vi "IPC-Core-UDPModule.vi"(8 "error in":errorcluster, 9 "ErrorQRef":refnum<queue>, 10 "DataQRef":refnum<queue>, 11 "UdpQRef":refnum<queue>) -> (0 "错误输出":errorcluster)   [LabVIEW 2014]
uses:
  Configuration-Global.vi
panel:
  out "数值 2":i32
  out "数值":i32
  in  "开关":bool=TRUE
  out "Udp::Initialize":string
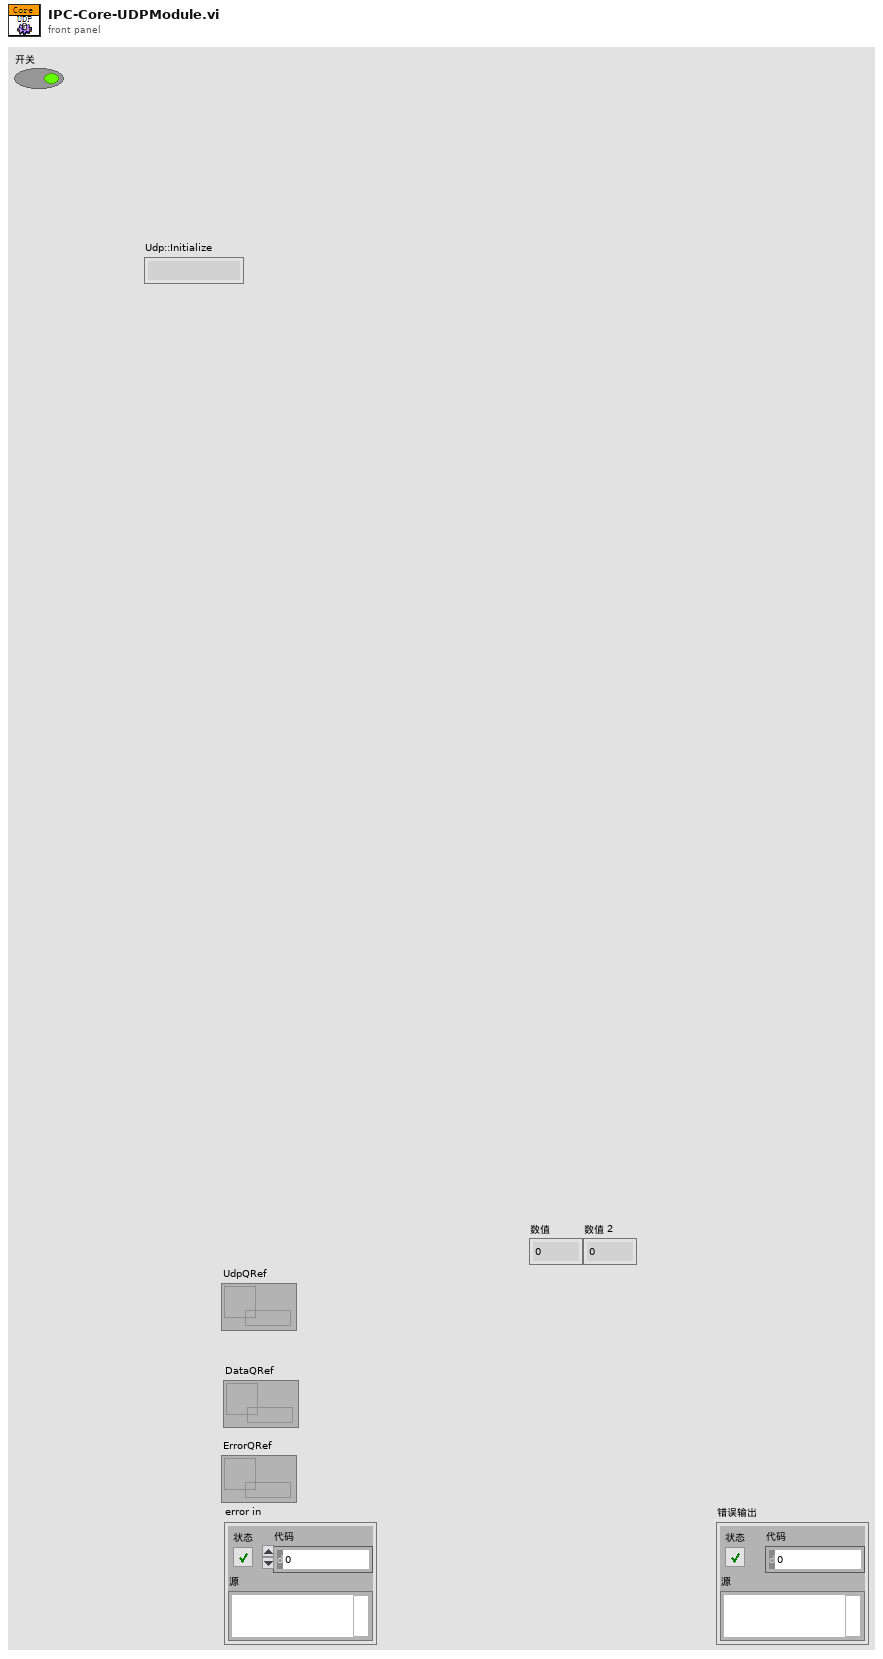
[diagram p1: front panel]
types:
  T1 = cluster{"时间":timestamp, "声发射":sgl[], "电涡流1":sgl[], "电涡流2":sgl[], "电涡流3":sgl[], "电涡流4":sgl[], "电涡流5":sgl[], "加速度1":sgl[], "加速度2":sgl[]}
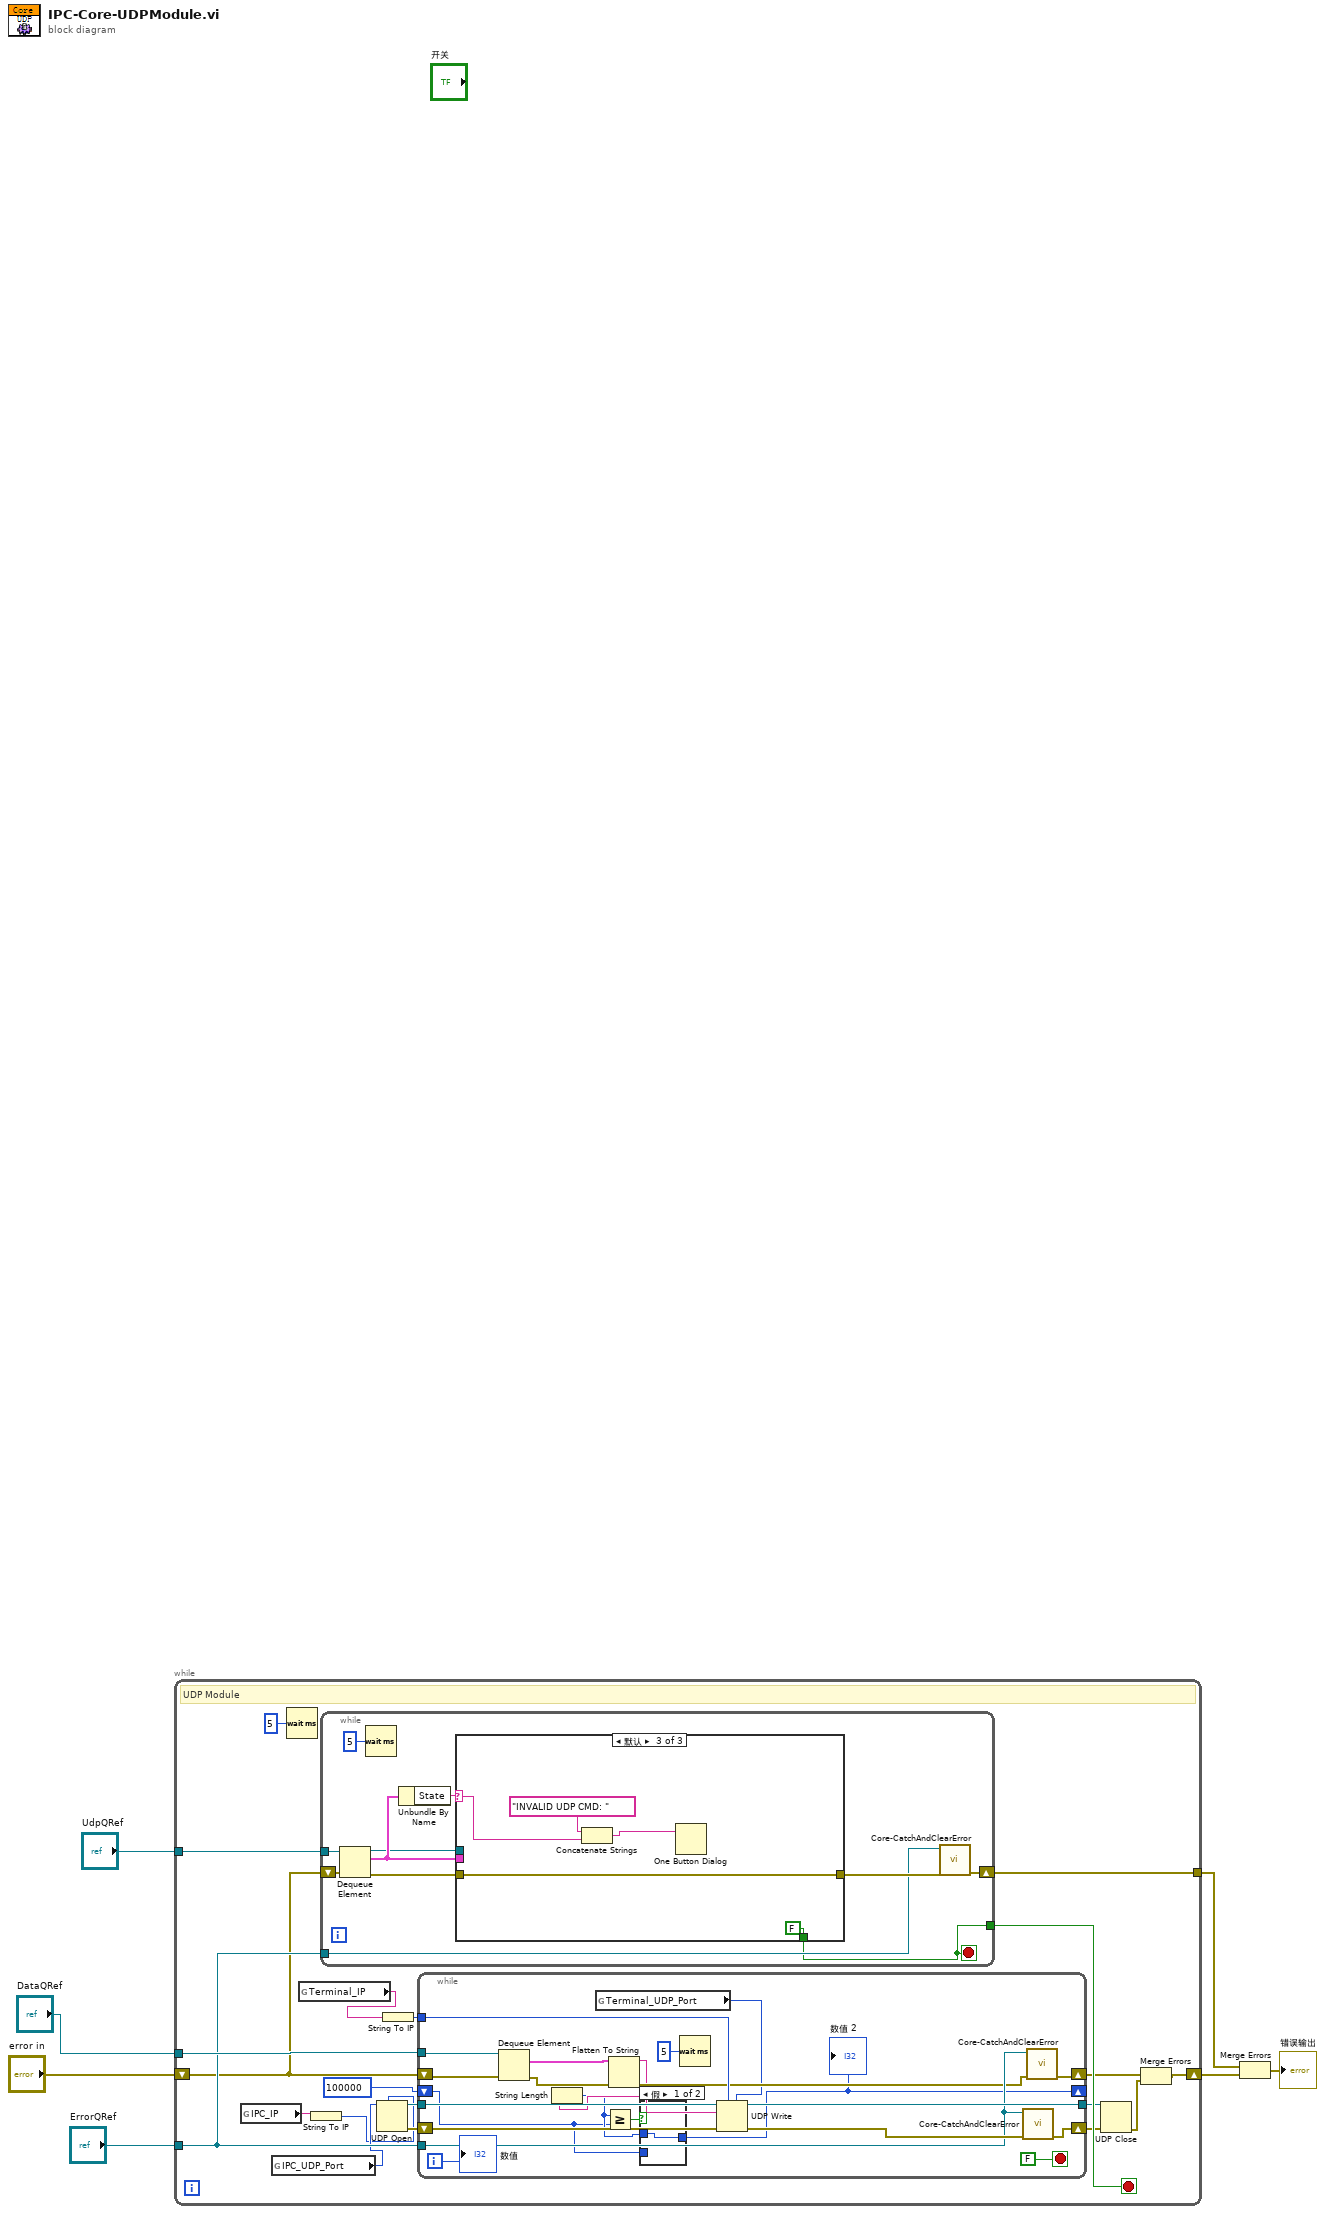
[diagram p0: block diagram]
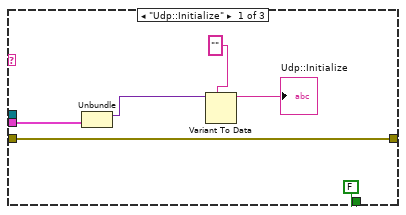
[diagram p3: hidden frame]
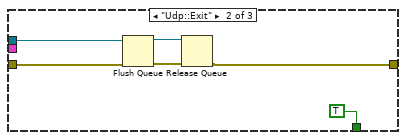
[diagram p4: hidden frame]
diagram:
  n1 = while {
    tunnel: "DataQRef" -> [w25]
    shift-right: [w13] -> w5
    shift-left: "error in" -> [w22]
    tunnel: "ErrorQRef" -> [w23]
    tunnel: "UdpQRef" -> [w26]
    tunnel: [w21] -> w4
    stop <- w24 stop-if-true
    # "UDP Module"
    n2 = global read "Configuration-Global.vi" "IPC_IP"() -> (w9:string)
    n3 = global read "Configuration-Global.vi" "IPC_UDP_Port"() -> (w11:i32)
    n4 = Wait (ms)(milliseconds to wait=u32 5 ("等待时间（毫秒）")) -> ()  [unwired: 1 out]
    n5 = global read "Configuration-Global.vi" "Terminal_IP"() -> (w10:string)
    n6 = String To IP(1:w9) -> (0:w8:u32)
    n7 = while {
      tunnel: w26 -> [w62]
      tunnel: [w53] -> w24
      tunnel: w23 -> [w54]
      shift-right: [w60] -> w21
      shift-left: w22 -> [w61]
      stop <- w53 stop-if-true
      n8 = Dequeue Element(queue=w62, error in (no error)=w61) -> (queue out=w55:refnum<queue>, element=w59:cluster{"Data":variant, "State":string}, error out=w57:errorcluster)  [unwired: 1 in, 1 out]
      n9 = Wait (ms)(milliseconds to wait=u32 5 ("等待时间（毫秒）")) -> ()  [unwired: 1 out]
      n10 = Unbundle By Name(w59) -> ("State"=w58:string)
      n11 = case shown="默认" w58 {
        selector: w58 -> [_ _ w77]
        tunnel: w59 -> [w66 _ _]
        tunnel: w57 -> [w68 w72 w76]
        tunnel: [w68 w71 w76] -> w56
        tunnel: w55 -> [_ w70 _]
        tunnel: [FALSE TRUE FALSE] -> w53
        frame "Udp::Initialize" {
          n12 = Unbundle(w66) -> ("Data"=w67:variant)  [unwired: 1 out]
          n13 = Variant To Data(type="", Variant=w67) -> (data=→"Udp::Initialize":string)  [unwired: 1 in, 1 out]
        }
        frame "Udp::Exit" {
          n14 = Flush Queue(queue=w70, error in (no error)=w72) -> (queue out=w74:refnum<queue>, error out=w73:errorcluster)  [unwired: 1 out]
          n15 = Release Queue(queue=w74, error in (no error)=w73) -> (error out=w71:errorcluster)  [unwired: 1 in, 2 out]
        }
        frame Default {
          n16 = Concatenate Strings("INVALID UDP CMD: ", w77) -> (w78:string)
          n17 = One Button Dialog(message=w78) -> ()  [unwired: 1 in, 1 out]
        }
      }
      n18 = call "Core-CatchAndClearError.vi"("error in (no error)"=w56, "ErrorQ"=w54) -> ("error out"=w60:errorcluster)  [unwired: 7 in]
    }
    n19 = UDP Open(7:w8, 11:w11) -> (port=w20:refnum<k16>, 0:w19:errorcluster)  [unwired: 3 in, 1 out]
    n20 = String To IP(1:w10) -> (0:w16:u32)
    n21 = while {
      tunnel: w23 -> [w38]
      tunnel: w25 -> [w48]
      shift-right: [w46] -> w14
      shift-left: w22 -> [w47]
      tunnel: w20 -> [w45]
      tunnel: [w43] -> w18
      shift-right: [w40] -> w17
      shift-left: w19 -> [w44]
      tunnel: w16 -> [w42]
      shift-right: [w29] -> _
      shift-left: 100000 -> [w30]
      i -> [w34]
      stop <- FALSE stop-if-true
      n22 = Dequeue Element(queue=w48, error in (no error)=w47) -> (element=w37:T1, error out=w36:errorcluster)  [unwired: 1 in, 2 out]
      n23 = global read "Configuration-Global.vi" "Terminal_UDP_Port"() -> (w28:i32)
      n24 = Flatten To String(anything=w37, error in (no error)=w36) -> (data string=w33:string, error out=w35:errorcluster)  [unwired: 2 in, 1 out]
      n25 = String Length(string=w33) -> (length=w31:i32)
      n26 = Greater Or Equal?(x=w31, y=w30) -> (x >= y?=w32:bool)
      n27 = case shown="假" w32 {
        tunnel: w31 -> [w50 _]
        tunnel: w30 -> [_ w51]
        tunnel: [w50 w51] -> w29
        frame False {
        }
        frame True {
        }
      }
      "数值 2" <- w29
      n28 = Wait (ms)(milliseconds to wait=u32 5 ("等待时间（毫秒）")) -> ()  [unwired: 1 out]
      n29 = UDP Write(address=w42, port or service name=w28, connection ID=w45, data in=w33, 8:w44) -> (error out=w39:errorcluster, 3:w43:refnum<k16>)  [unwired: 1 in]
      n30 = call "Core-CatchAndClearError.vi"("error in (no error)"=w39, "ErrorQ"=w38) -> ("error out"=w40:errorcluster)  [unwired: 7 in]
      n31 = call "Core-CatchAndClearError.vi"("error in (no error)"=w35, "ErrorQ"=w38) -> ("error out"=w46:errorcluster)  [unwired: 7 in]
      "数值" <- w34
    }
    n32 = UDP Close(connection ID=w18, 8:w17) -> (error out=w15:errorcluster)  [unwired: 1 out]
    n33 = Merge Errors(w14, w15) -> (w13:errorcluster)
  }
  n34 = Merge Errors(w4, w5) -> (→"错误输出":errorcluster)
